vi "Read Control.vi"(0 "VI Name":string="Untitled 1.vi", 1 "Control Name":string="Numeric", 2 "Target LV Version #":T1, 3 "Machine Name":string, 4 "vi reference":refnum<vi>) -> (5 "Value":variant, 6 "error out":errorcluster)   [LabVIEW 2020]
uses:
  Sub Controls/LV Versions Enum.ctl
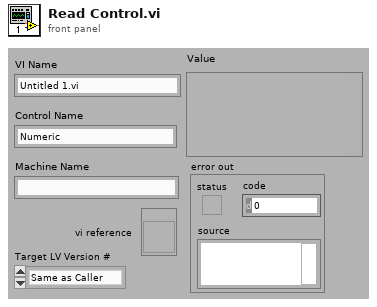
[diagram p1: front panel]
types:
  T1 = typedef "LV Versions Enum.ctl" = enum16{"Same as Caller", "8.0", "8.20", "8.5", "8.6", "9.0", "10.0", "11.0", "12.0", "13.0", "14.0", "15.0", "16.0", "17.0", "18.0", "19.0", "20.0"}
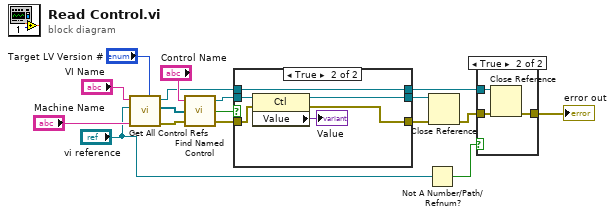
[diagram p0: block diagram]
diagram:
  n1 = call "Get All Control Refs.vi"("VI Name"="VI Name", "vi reference"="vi reference", "Machine Name"="Machine Name", "Target LV Version #"="Target LV Version #") -> ("VI Refnum"=w7:refnum<vi>, "All Controls"=w10:refnum<vi>[], "error out"=w11:errorcluster)  [unwired: 2 in]
  n2 = call "Find Named Control.vi"("error in"=w11, "All Controls"=w10, "Control Name"="Control Name") -> ("error out"=w12:errorcluster, "Found"=w16:bool, "Ctl Refnum"=w15:refnum<vi>)
  n3 = case shown="True" w16 {
    tunnel: w15 -> [w19 w26]
    tunnel: [w19 w25] -> w14
    tunnel: [w20 w24] -> w13
    tunnel: w12 -> [w20 w23]
    tunnel: w7 -> [w18 w22]
    tunnel: [w18 w22] -> w6
    frame False {
    }
    frame True {
      n4 = property class="Ctl"(reference=w26, error in=w23) -> (reference out=w25:refnum<vi>, error out=w24:errorcluster, "Value"=→"Value":variant)
    }
  }
  n5 = Not A Number/Path/Refnum?(number/path/refnum="vi reference") -> (NaN/Path/Refnum?=w3:bool)
  n6 = Close Reference(reference=w14, error in (no error)=w13) -> (error out=w5:errorcluster)
  n7 = case shown="True" w3 {
    tunnel: w6 -> [_ w30]
    tunnel: w5 -> [w27 w29]
    tunnel: [w27 w28] -> w4
    frame False {
    }
    frame True {
      n8 = Close Reference(reference=w30, error in (no error)=w29) -> (error out=w28:errorcluster)
    }
  }
  "error out" <- w4
